vi "RSZVB Set Marker Search Mode.vi"(7 "Search Mode (0: Bandpass Ref to Max)":i32(ring) items=["Bandpass Ref to Max", "Bandstop Ref to Max", "Bandpass Ref to Marker", "Bandstop Ref to Marker", "Bandpass Absolute Level", "Bandstop Absolute Level"], 8 "error in (no error)":errorcluster {"code" format="%.0x"}, 9 "Marker (1)":i32=1, 10 "Channel (Trace) (1)":i32=1, 11 "VISA session":refnum<visa-resource-name>) -> (0 "error out":errorcluster {"code" format="%.0x"}, 3 "dup VISA session":refnum<visa-resource-name>)   [LabVIEW 2011]
doc: "This VI selects the bandfilter search mode.\n\nRemote-control command(s):\nCALCulate<Chn>:MARKer<Mk>:FUNCtion:BWIDth:MODE\nBPASs | BSTop | BPRMarker | BSRMarker | BPABsolute | BSABsolute"
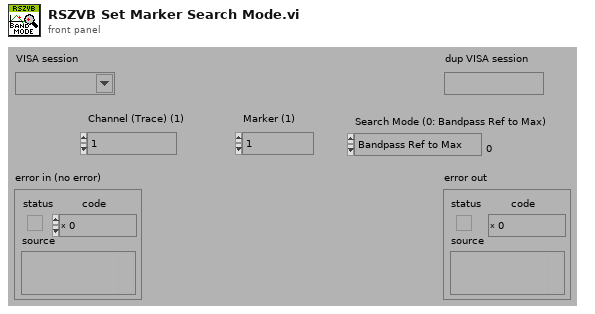
[diagram p1: front panel]
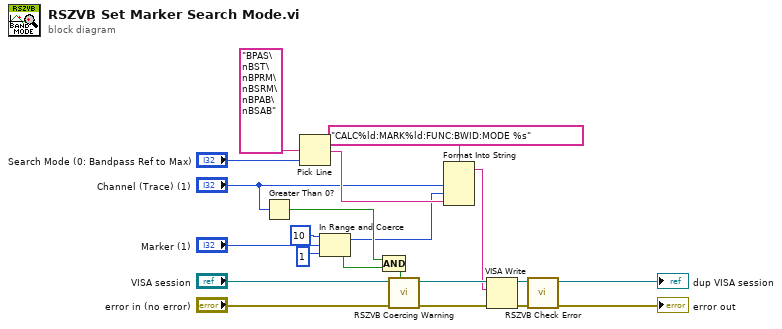
[diagram p0: block diagram]
diagram:
  n1 = Greater Than 0?(x="Channel (Trace) (1)") -> (x > 0?=w4:bool)
  n2 = Pick Line(multi-line string="BPAS\nBST\nBPRM\nBSRM\nBPAB\nBSAB", line index="Search Mode (0: Bandpass Ref to Max)") -> (output string=w5:string)  [unwired: 1 in]
  n3 = In Range and Coerce(upper limit=10, x="Marker (1)", lower limit=1) -> (coerced(x)=w1:i32, In Range?=w3:bool)
  n4 = Compound Arithmetic op=AND(w4, w3) -> (w14:bool)
  n5 = call "RSZVB Coercing Warning.vi"("In Range?"=w14, "error in (no error)"="error in (no error)", "VISA session"="VISA session") -> ("error out"=w20:errorcluster, "dup VISA session"=w21:refnum<visa-resource-name>)  [unwired: 7 in]
  n6 = Format Into String(format string="CALC%ld:MARK%ld:FUNC:BWID:MODE %s", "Channel (Trace) (1)", w1, w5) -> (resulting string=w13:string)  [unwired: 2 in, 1 out]
  n7 = VISA Write(VISA resource name=w21, write buffer=w13, error in (no error)=w20) -> (VISA resource name out=w18:refnum<visa-resource-name>, error out=w19:errorcluster)  [unwired: 1 out]
  n8 = call "RSZVB Check Error.vi"("error in (no error)"=w19, "VISA session"=w18) -> ("error out"=→"error out":errorcluster, "dup VISA session"=→"dup VISA session":refnum<visa-resource-name>)  [unwired: 8 in]
